vi "ErrorHandler.vi"(4 "Local Event":string, 6 "Local Event":refnum<queue>, 7 "Global_Event":refnum<user-event>, 8 "error in":errorcluster) -> (0 "error out":errorcluster)   [LabVIEW 2013]
panel:
  out "Error Log":T1(array[cluster])
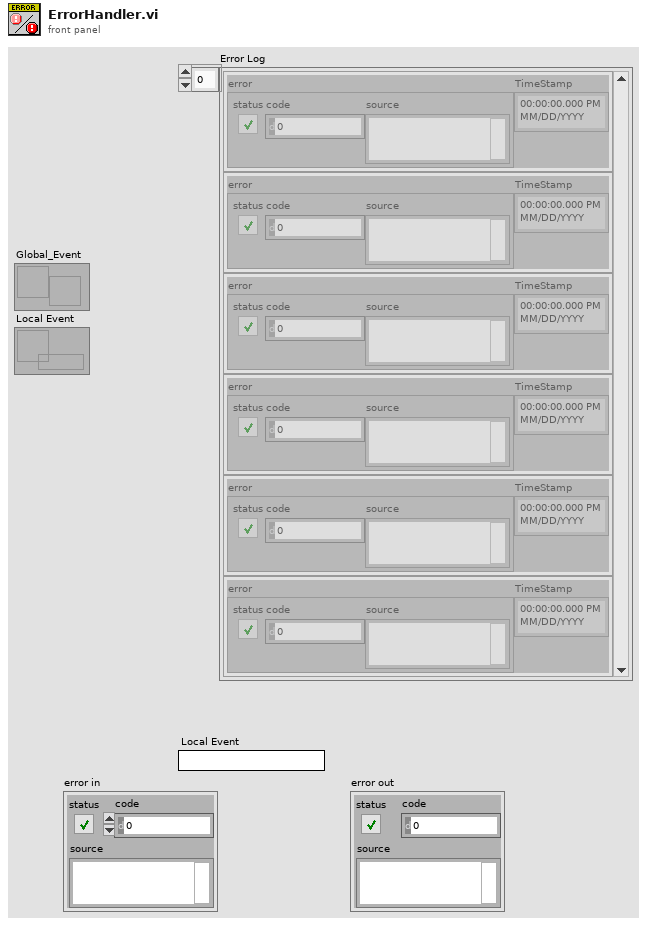
[diagram p1: front panel]
types:
  T1 = cluster{"error":errorcluster, "TimeStamp":timestamp}[]
  T2 = enum32{"Invalid", "Standard", "Closed", "Hidden", "Minimized", "Maximized"}
  T3 = cluster{"error":errorcluster, "TimeStamp":timestamp}
  T4 = typedef "ErrorHandler_OBJ - PROP.ctl" = cluster{"Log?":bool, "DefaultAction":enum16{"Clear", "Continue"}, "actions":cluster{"code":i32, "Action":enum16{"Clear", "Continue"}, "GLB_Event":string, "Local_Event":string}[], "errorLog":cluster{"error":errorcluster, "TimeStamp":timestamp}[], "writeLog?":bool, "logPath":path}
  T5 = cluster{"code":i32, "Action":enum16{"Clear", "Continue"}, "GLB_Event":string, "Local_Event":string}[]
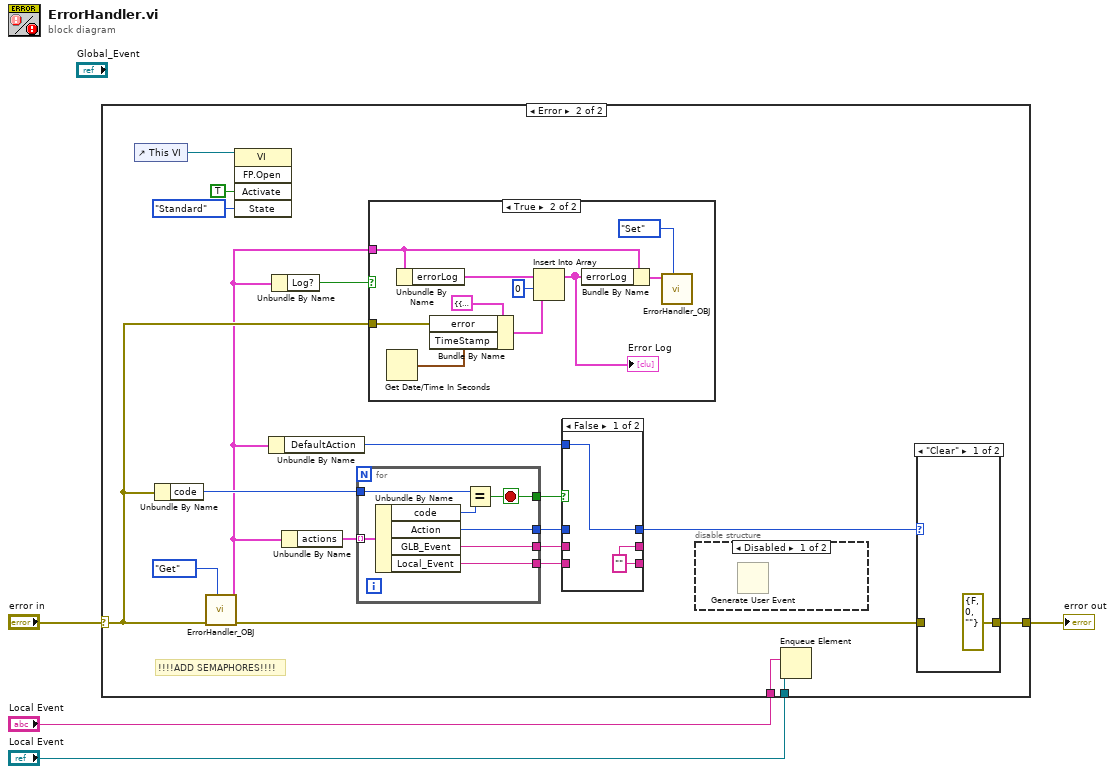
[diagram p0: block diagram]
diagram:
  n1 = case shown="Error" "error in" {
    selector: "error in" -> [w5 w22]
    tunnel: [w5 w11] -> w3
    tunnel: "Local Event" -> [_ w10]
    tunnel: "Local Event" -> [_ w9]
    frame No Error {
    }
    frame Error {
      # "!!!!ADD SEMAPHORES!!!!"
      n2 = control-ref of="This VI"() -> (w8:refnum<vi>)
      n3 = Unbundle By Name(w22) -> ("code"=w20:i32)
      n4 = call "ErrorHandler_OBJ.vi"("Mode"=enum16{"Get", "Set"}."Get", "error in"=w22) -> ("error out"=w13:errorcluster, "PROPERTIES OUT"=w19:T4)  [unwired: 8 in]
      n5 = invoke class="VI" method="FP.Open"(reference=w8, "Activate"=TRUE ("Activate?"), "State"=T2."Standard") -> ()  [unwired: 2 in, 5 out]
      n6 = Unbundle By Name(w19) -> ("DefaultAction"=w14:enum16{"Clear", "Continue"})
      n7 = Unbundle By Name(w19) -> ("Log?"=w23:bool)
      n8 = Unbundle By Name(w19) -> ("actions"=w21:T5)
      n9 = for {
        tunnel: w21 -> [w38] mode=indexing
        tunnel: w20 -> [w37]
        tunnel: [w35] -> w18
        tunnel: [w34] -> w17
        tunnel: [w33] -> w16
        tunnel: [w32] -> w15
        stop <- w35 stop-if-true
        n10 = Unbundle By Name(w38) -> ("code"=w36:i32, "Action"=w34:enum16{"Clear", "Continue"}, "GLB_Event"=w33:string, "Local_Event"=w32:string)
        n11 = Equal?(x=w37, y=w36) -> (x = y?=w35:bool)
      }
      n12 = case shown="True" w23 {
        tunnel: w19 -> [_ w47]
        tunnel: w22 -> [_ w41]
        frame False {
        }
        frame True {
          n13 = Get Date/Time In Seconds() -> (seconds since 1Jan1904=w39:timestamp)
          n14 = Unbundle By Name(w47) -> ("errorLog"=w44:T1)
          n15 = Bundle By Name(cluster=T3 {"error"={"status"=FALSE, "code"=0, "source"=""}, "TimeStamp"=timestamp(0 s since 1904-01-01)} ("Cluster"), "error"=w41, "TimeStamp"=w39) -> (w40:T3)
          n16 = Insert Into Array(array=w44, index=0, new element=w40) -> (w43:T1)
          "Error Log" <- w43
          n17 = Bundle By Name(cluster=w47, "errorLog"=w43) -> (w46:T4)
          n18 = call "ErrorHandler_OBJ.vi"("Mode"=enum16{"Get", "Set"}."Set", "PROPERTIES IN"=w46) -> ()  [unwired: 8 in, 2 out]
        }
      }
      n19 = case shown="False" w18 {
        tunnel: w17 -> [_ w31]
        tunnel: [w28 w31] -> w12
        tunnel: w16 -> [_ w30]
        tunnel: w15 -> [_ w29]
        tunnel: [w27 w30] -> _
        tunnel: [w27 w29] -> _
        tunnel: w14 -> [w28 _]
        frame False {
          w27 = "" ("Local_Event")
        }
        frame True {
        }
      }
      n20 = disable-structure shown="Disabled" {
        frame Disabled {
          n21 = Generate User Event() -> ()  [unwired: 4 in, 2 out]
        }
        frame Enabled {
        }
      }
      n22 = Enqueue Element(queue=w10, element=w9) -> ()  [unwired: 2 in, 3 out]
      n23 = case shown="\"Clear\"" w12 {
        tunnel: w13 -> [_ w26]
        tunnel: [errorcluster {"status"=FALSE, "code"=0, "source"=""} ("error out") w26] -> w11
        frame "Clear" {
        }
        frame "Continue" {
        }
      }
    }
  }
  "error out" <- w3
